vi "coulbourn-sound.vi"() -> ()   [LabVIEW 2013]
panel:
  in  "Digital DAQ Channel":tag
  in  "Save Session Stim List":bool
  in  "Sound DAQ Channel":tag
  out "Runtime Errors":errorcluster
  out "Current (or Cued) Waveform":dbl[](graph)
  out "Playing Stimulus":bool caption="Playing stimulus"
  in  "Current (or Cued) Trial":i32(slide) scale=0.0..60.0
  out "Waiting for trigger":bool
  out "Stimulus List File Path":path
  in  "Load Session Stim List":bool
  out "Trial Parameters File Path":path
  in  "Load Trial Param":bool
  in  "Save Trial Param":bool
  in  "Trial Randomization":enum32{"50% exactly", "Radio Selection 2"}(radio)
  in  "NoGo Stims":dbl[][](array[numeric])
  in  "Total Trials":i32=60 min=2
  in  "Go Stims":dbl[][](array[numeric])
  out "Stimulus List":dbl[][](array[numeric])
  in  "Play Session Stim List":bool
  in  "Generate Trial Stim List":bool
  # "Stim Code, Stim Type, Duration, Param 1, Param 2, Param 3, Param 4"
  # "Stim Code, Stim Type, Duration, Param 1, Param 2, Param 3, Param 4"
  # "GONOGO, Stim Code, Stim Type, Duration, Param 1, Param 2, Param 3, Param 4"
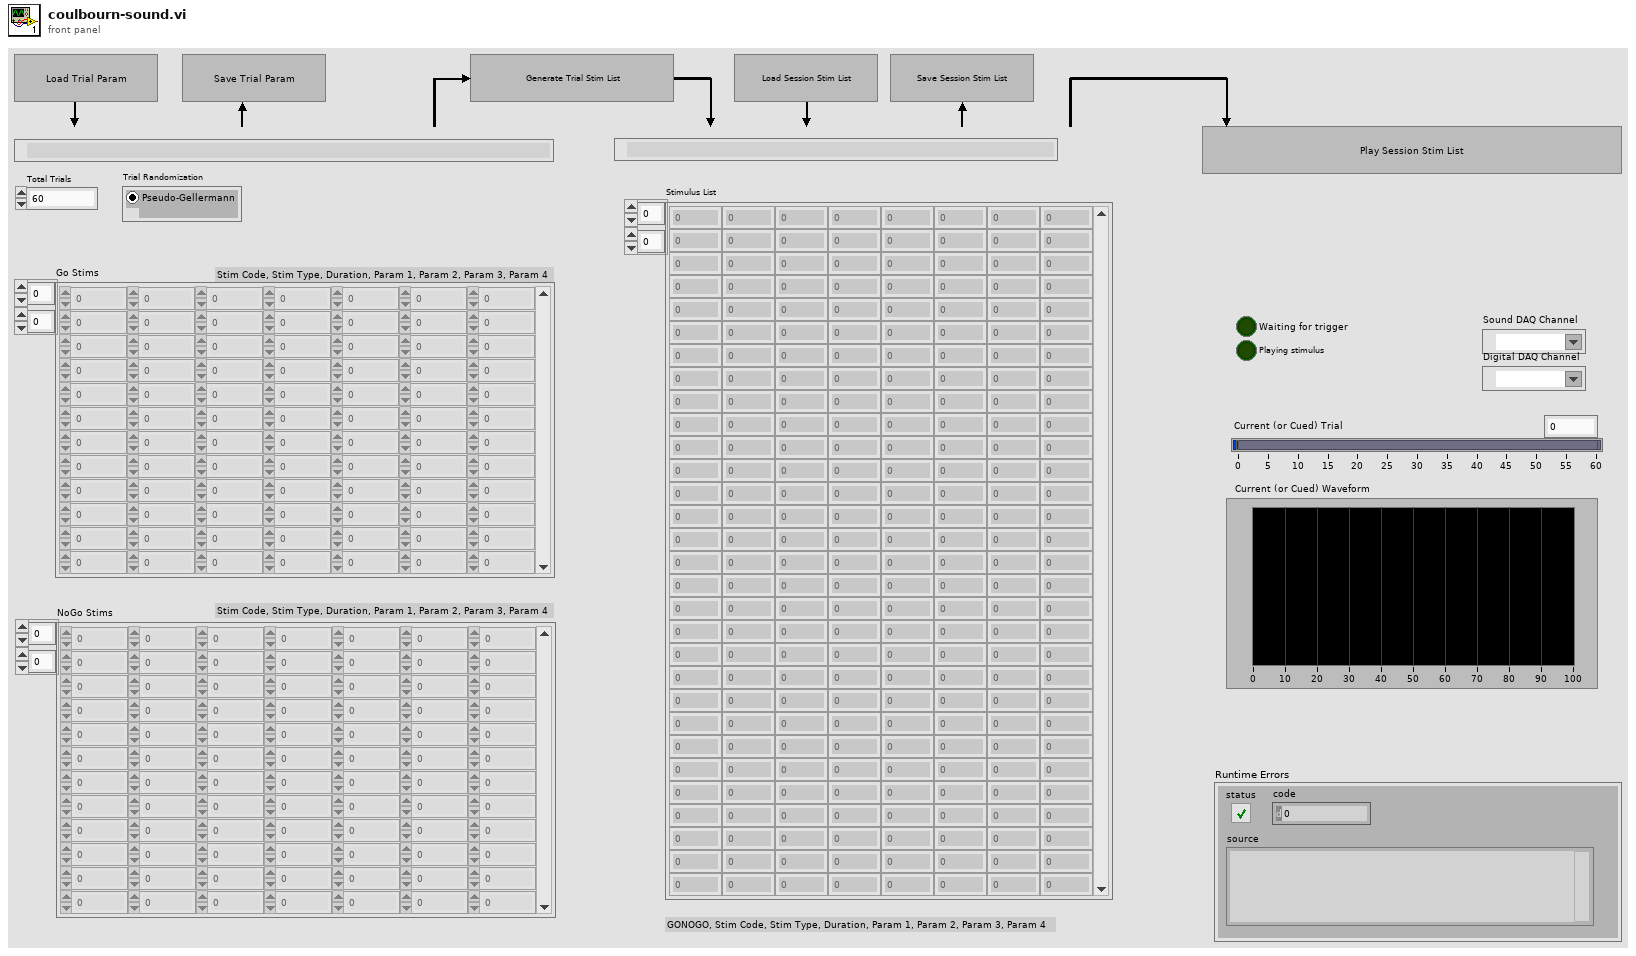
[diagram p1: front panel]
types:
  T1 = enum8{"Enabled", "Disabled", "Disabled and Grayed Out"}
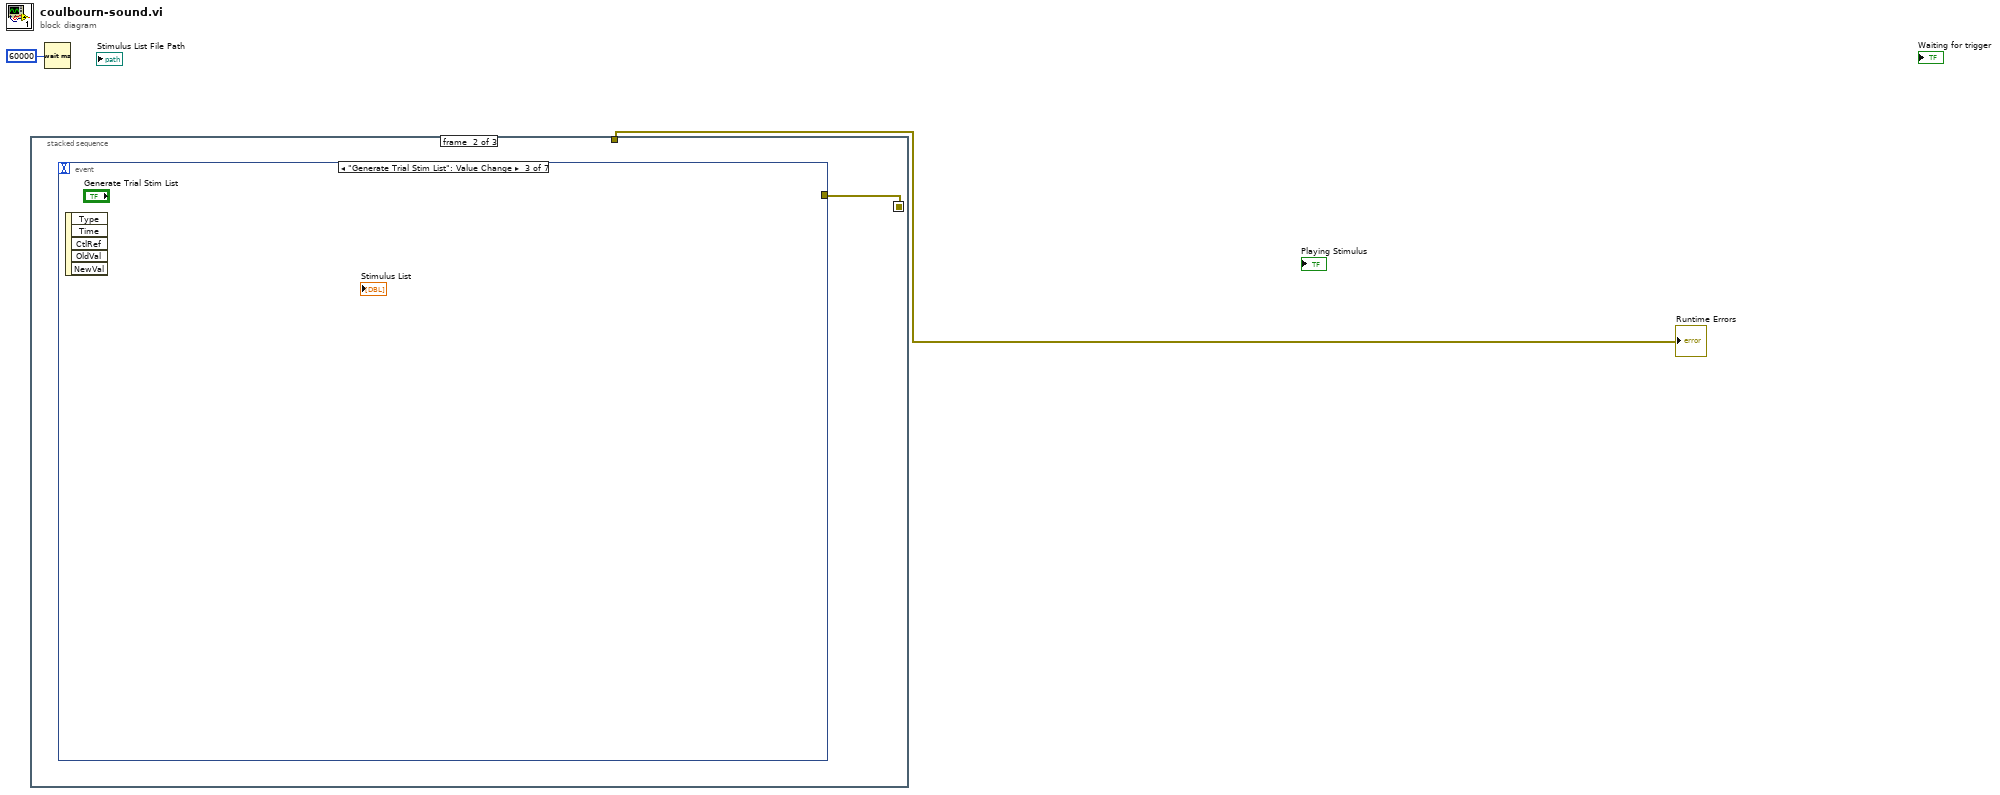
[diagram p0: block diagram]
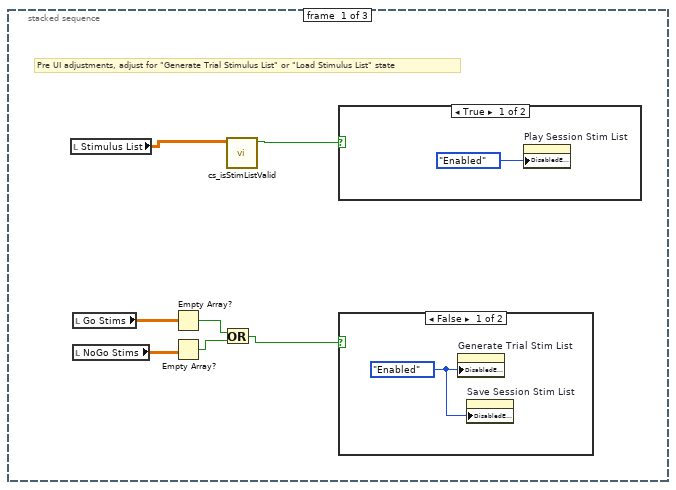
[diagram p2: hidden frame]
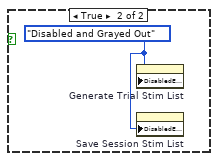
[diagram p3: hidden frame]
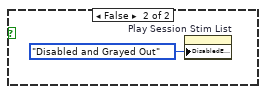
[diagram p4: hidden frame]
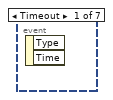
[diagram p5: hidden frame]
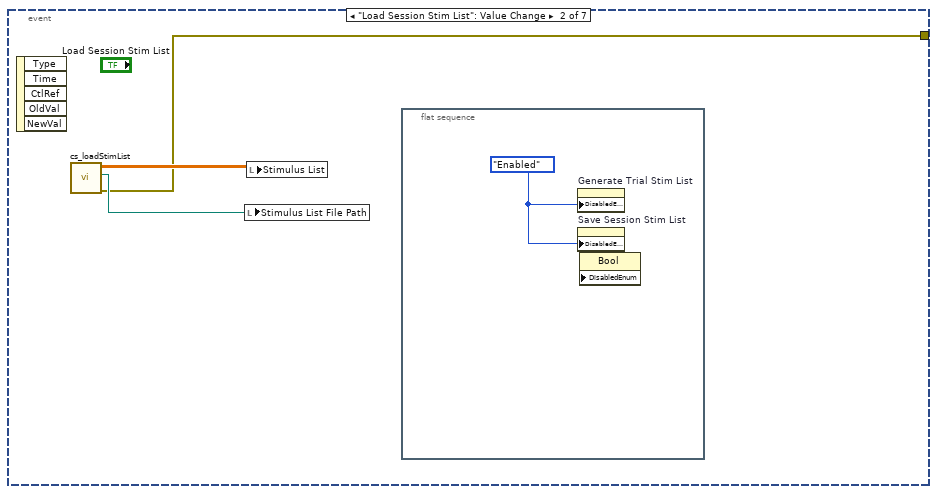
[diagram p6: hidden frame]
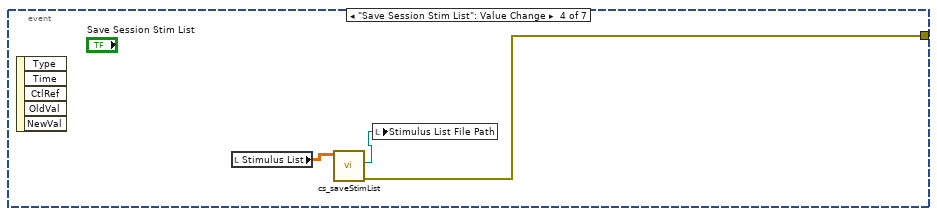
[diagram p7: hidden frame]
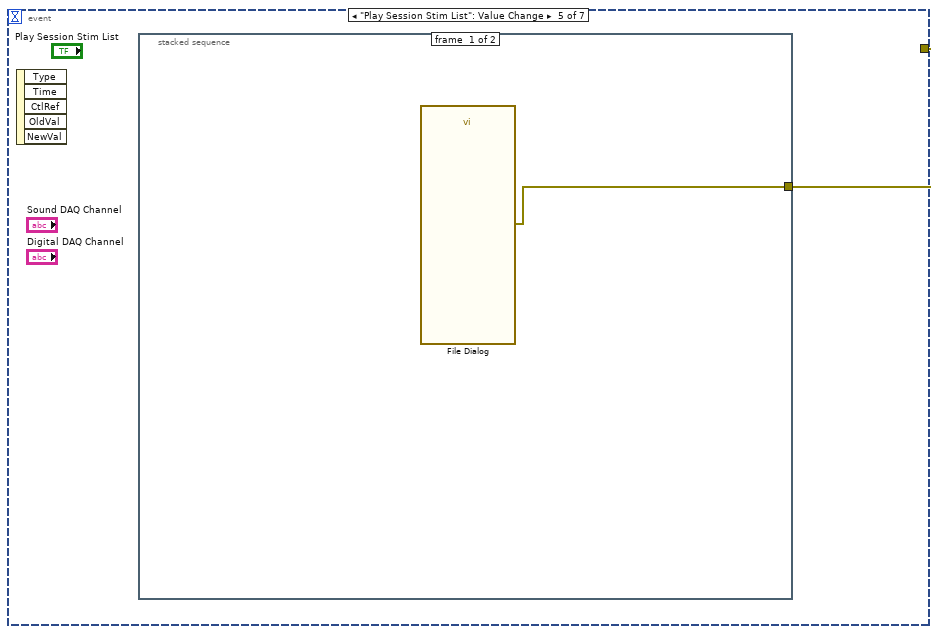
[diagram p8: hidden frame]
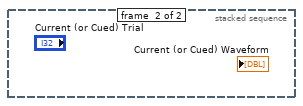
[diagram p9: hidden frame]
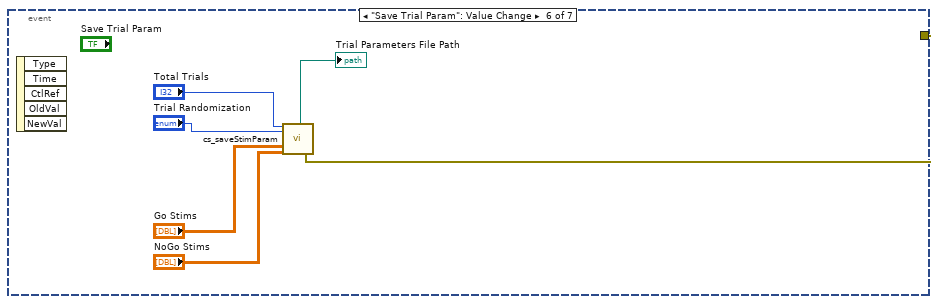
[diagram p10: hidden frame]
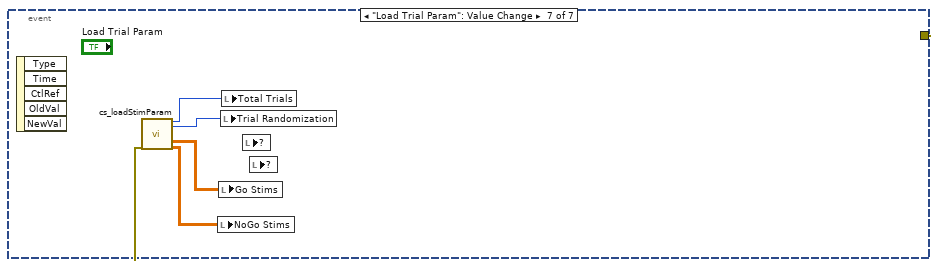
[diagram p11: hidden frame]
diagram:
  n1 = stacked-sequence {
    seq-local: [_ w14 _] -> [_ _ w35]
    tunnel: [_ _ w35] -> w1
    frame #0 {
      # "Pre UI adjustments, adjust for \"Generate Trial Stimulus List\" or \"Load Stimulus List\" state"
      n2 = local read "Stimulus List"() -> (w4:dbl[][])
      n3 = local read "Go Stims"() -> (w8:dbl[][])
      n4 = local read "NoGo Stims"() -> (w9:dbl[][])
      n5 = Empty Array?(array=w8) -> (empty?=w7:bool)
      n6 = Empty Array?(array=w9) -> (empty?=w6:bool)
      n7 = Or(x=w7, y=w6) -> (x .or. y?=w5:bool)
      n8 = call "cs_isStimListValid.vi"("Array"=w4) -> ("Valid?"=w3:bool)  [unwired: 9 in, 1 out]
      n9 = case shown="True" w3 {
        frame True {
          n10 = property on="Play Session Stim List" class="Bool"("DisabledEnum"=T1."Enabled" ("Disabled")) -> ()  [unwired: 2 in, 2 out]
        }
        frame False {
          n11 = property on="Play Session Stim List" class="Bool"("DisabledEnum"=T1."Disabled and Grayed Out" ("Disabled")) -> ()  [unwired: 2 in, 2 out]
        }
      }
      n12 = case shown="False" w5 {
        frame False {
          w10 = T1."Enabled" ("Disabled")
          n13 = property on="Generate Trial Stim List" class="Bool"("DisabledEnum"=w10) -> ()  [unwired: 2 in, 2 out]
          n14 = property on="Save Session Stim List" class="Bool"("DisabledEnum"=w10) -> ()  [unwired: 2 in, 2 out]
        }
        frame True {
          w11 = T1."Disabled and Grayed Out" ("Disabled")
          n15 = property on="Generate Trial Stim List" class="Bool"("DisabledEnum"=w11) -> ()  [unwired: 2 in, 2 out]
          n16 = property on="Save Session Stim List" class="Bool"("DisabledEnum"=w11) -> ()  [unwired: 2 in, 2 out]
        }
      }
    }
    frame #1 {
      n17 = event shown="[2] \"Generate Trial Stim List\": Value Change" {
        selector: _ -> [_ _ _ _ _ _ _]
        dyn-events: _ -> [_ _ _ _ _ _ _]
        timeout: _ -> [_ _ _ _ _ _ _]
        tunnel: [_ w15 _ w19 w22 w24 w30] -> w14
        event Timeout {
          n18 = event-data() -> ()  [unwired: 1 in, 2 out]
        }
        event "Load Session Stim List": Value Change {
          n19 = event-data() -> ()  [unwired: 1 in, 5 out]
          n20 = call "cs_loadStimList.vi"() -> ("error out"=w15:errorcluster, "Path"=w16:path, "Stimulus List"=w17:dbl[][])  [unwired: 5 in]
          n21 = local write "Stimulus List File Path"(w16) -> ()
          n22 = local write "Stimulus List"(w17) -> ()
          n23 = flat-sequence {
            frame #0 {
              w18 = T1."Enabled" ("Disabled")
              n24 = property on="Generate Trial Stim List" class="Bool"("DisabledEnum"=w18) -> ()  [unwired: 2 in, 2 out]
              n25 = property on="Save Session Stim List" class="Bool"("DisabledEnum"=w18) -> ()  [unwired: 2 in, 2 out]
              n26 = property on="Property Node" class="Bool" props=["DisabledEnum"]() -> ()  [unwired: 3 in, 2 out]
            }
          }
        }
        event "Generate Trial Stim List": Value Change {
          n27 = event-data() -> ()  [unwired: 1 in, 5 out]
        }
        event "Save Session Stim List": Value Change {
          n28 = event-data() -> ()  [unwired: 1 in, 5 out]
          n29 = local read "Stimulus List"() -> (w20:dbl[][])
          n30 = call "cs_saveStimList.vi"("Stimulus List"=w20) -> ("error out"=w19:errorcluster, "Path"=w21:path)  [unwired: 5 in]
          n31 = local write "Stimulus List File Path"(w21) -> ()
        }
        event "Play Session Stim List": Value Change {
          n32 = event-data() -> ()  [unwired: 1 in, 5 out]
          n33 = stacked-sequence {
            tunnel: [w23 _] -> w22
            frame #0 {
              n34 = call "File Dialog"() -> ("error out"=w23:errorcluster)  [unwired: 12 in, 3 out]
            }
            frame #1 {
            }
          }
        }
        event "Save Trial Param": Value Change {
          n35 = event-data() -> ()  [unwired: 1 in, 5 out]
          n36 = call "cs_saveStimParam.vi"("Total Trials"="Total Trials", "Trial Randomization"="Trial Randomization", "Stims 1"="Go Stims", "Stims 2"="NoGo Stims") -> ("Path"=→"Trial Parameters File Path":path, "error out"=w24:errorcluster)  [unwired: 14 in]
        }
        event "Load Trial Param": Value Change {
          n37 = event-data() -> ()  [unwired: 1 in, 5 out]
          n38 = call "cs_loadStimParam.vi"() -> ("error out"=w30:errorcluster, "Total Trials"=w34:i32, "Trial Randomization"=w33:enum32{"50% exactly", "Radio Selection 2"}, "Stims 1"=w32:dbl[][], "Stims 2"=w31:dbl[][])  [unwired: 12 in, 3 out]
          n39 = local write "NoGo Stims"(w31) -> ()
          n40 = local write "Go Stims"(w32) -> ()
          n41 = local write "Trial Randomization"(w33) -> ()
          n42 = local write "Total Trials"(w34) -> ()
          n43 = local read item#-1() -> ()  [unwired: 1 in]
          n44 = local read item#-1() -> ()  [unwired: 1 in]
        }
      }
    }
    frame #2 {
      # "Post UI Adjustments"
    }
  }
  "Runtime Errors" <- w1
  n45 = Wait (ms)(milliseconds to wait=u32 60000) -> ()  [unwired: 1 out]
